vi "Kinesis Move.vi"(8 "error in (no error)":errorcluster, 10 "Move Position":dbl, 11 ".NET Refnum in":refnum<k24>) -> (0 "error out":errorcluster, 3 "Position":dbl)   [LabVIEW 2023]
uses:
  E:/Old PC/desktop/Sensitive EQE Stuff/S-EQE (YJ)/Current Version/Thorlabs.MotionControl.Benchtop.StepperMotorCLI.dll
  Current Version/Thorlabs.MotionControl.Benchtop.StepperMotorCLI.dll
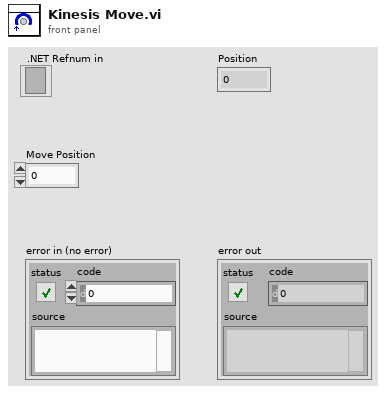
[diagram p1: front panel]
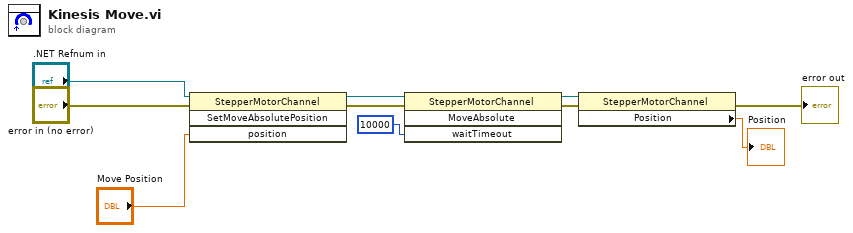
[diagram p0: block diagram]
diagram:
  n1 = invoke class="StepperMotorChannel" method="SetMoveAbsolutePosition"(reference=".NET Refnum in", error in="error in (no error)", "position"="Move Position") -> (reference out=w2:refnum<k24>, error out=w7:errorcluster)  [unwired: 1 in, 2 out]
  n2 = invoke class="StepperMotorChannel" method="MoveAbsolute"(reference=w2, error in=w7, "waitTimeout"=10000) -> (reference out=w9:refnum<k24>, error out=w10:errorcluster)  [unwired: 1 in, 2 out]
  n3 = property class="StepperMotorChannel"(reference=w9, error in=w10) -> (error out=→"error out":errorcluster, "Position"=→"Position":dbl)  [unwired: 1 out]
